vi "Test Serial.vi"() -> ()   [LabVIEW 2015]
uses:
  <vilib>/eio/EIOMethodNode/EIOMethodNode.xnode
  <vilib>/rvi/eio/common/nirviEmuTemplateMethod_errors.vi
  RS485 In.ctl
  Port.ctl
panel:
  out "Output":T1={"Data"=[0, 0, 0, 0, 0, 0, 0, 0, 0, 0, 0, 0, 0, 0, 0, 0, 0, 0, 0, 0, 0, 0, 0, 0, 0, 0, 0, 0, 0, 0, 0, 0, 0, 0, 0, 0, 0, 0, 0, 0, 0, 0, 0, 0, 0, 0, 0, 0, 0, 0, 0, 0, 0, 0, 0, 0, 0, 0, 0, 0, 0, 0, 0, 0, 0, 0, 0, 0, 0, 0, 0, 0, 0, 0, 0, 0, 0, 0, 0, 0, 0, 0, 0, 0, 0, 0, 0, 0, 0, 0, 0, 0, 0, 0, 0, 0, 0, 0, 0, 0, 0, 0, 0, 0, 0, 0, 0, 0, 0, 0, 0, 0, 0, 0, 0, 0, 0, 0, 0, 0, 0, 0, 0, 0, 0, 0, 0, 0, 0, 0, 0, 0, 0, 0, 0, 0, 0, 0, 0, 0, 0, 0, 0, 0, 0, 0, 0, 0, 0, 0, 0, 0, 0, 0, 0, 0, 0, 0, 0, 0, 0, 0, 0, 0, 0, 0, 0, 0, 0, 0, 0, 0, 0, 0, 0, 0, 0, 0, 0, 0, 0, 0, 0, 0, 0, 0, 0, 0, 0, 0, 0, 0, 0, 0, 0, 0, 0, 0, 0, 0], "NumBytes"=0, "RS485_Cmd"=enum."Read", "Port"=enum."Port 1", "Timeout (ms)"=0, "New"=FALSE}
  in  "Input":T1={"Data"=[0, 0, 0, 0, 0, 0, 0, 0, 0, 0, 0, 0, 0, 0, 0, 0, 0, 0, 0, 0, 0, 0, 0, 0, 0, 0, 0, 0, 0, 0, 0, 0, 0, 0, 0, 0, 0, 0, 0, 0, 0, 0, 0, 0, 0, 0, 0, 0, 0, 0, 0, 0, 0, 0, 0, 0, 0, 0, 0, 0, 0, 0, 0, 0, 0, 0, 0, 0, 0, 0, 0, 0, 0, 0, 0, 0, 0, 0, 0, 0, 0, 0, 0, 0, 0, 0, 0, 0, 0, 0, 0, 0, 0, 0, 0, 0, 0, 0, 0, 0, 0, 0, 0, 0, 0, 0, 0, 0, 0, 0, 0, 0, 0, 0, 0, 0, 0, 0, 0, 0, 0, 0, 0, 0, 0, 0, 0, 0, 0, 0, 0, 0, 0, 0, 0, 0, 0, 0, 0, 0, 0, 0, 0, 0, 0, 0, 0, 0, 0, 0, 0, 0, 0, 0, 0, 0, 0, 0, 0, 0, 0, 0, 0, 0, 0, 0, 0, 0, 0, 0, 0, 0, 0, 0, 0, 0, 0, 0, 0, 0, 0, 0, 0, 0, 0, 0, 0, 0, 0, 0, 0, 0, 0, 0, 0, 0, 0, 0, 0, 0], "NumBytes"=0, "RS485_Cmd"=enum."Idle", "Port"=enum."Port 1", "Timeout (ms)"=0, "New"=FALSE}
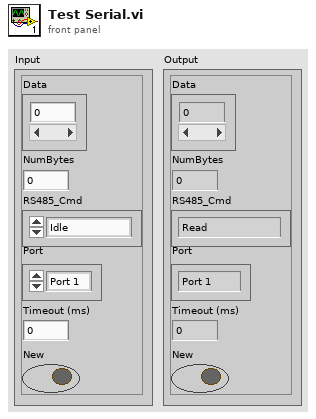
[diagram p1: front panel]
types:
  T1 = typedef "RS485 In.ctl" = cluster{"Data":u8[], "NumBytes":i32, "RS485_Cmd":enum8{"Read", "Write", "Idle"}, "Port":T2, "Timeout (ms)":i32, "New":bool}
  T2 = typedef "Port.ctl" = enum8{"Port 1", "Port 2", "Port 3", "Port 4", "None"}
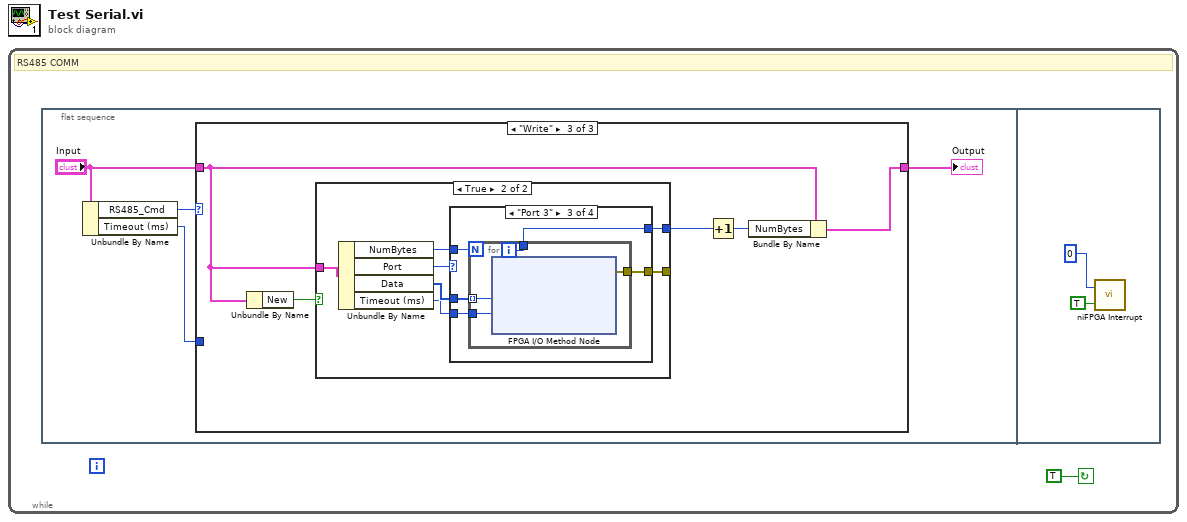
[diagram p0: block diagram]
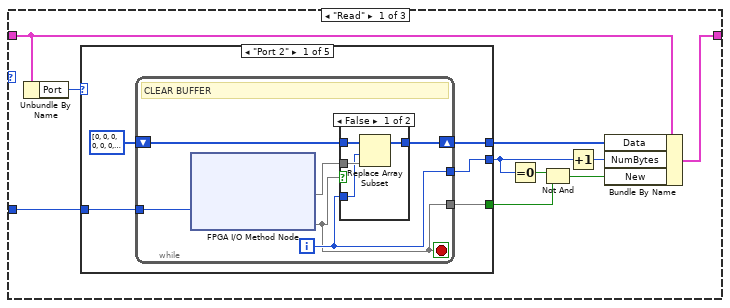
[diagram p2: hidden frame]
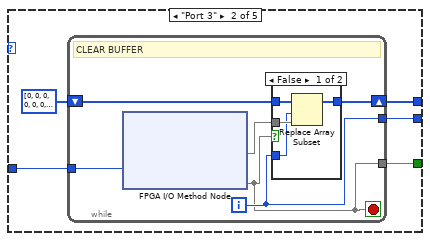
[diagram p4: hidden frame]
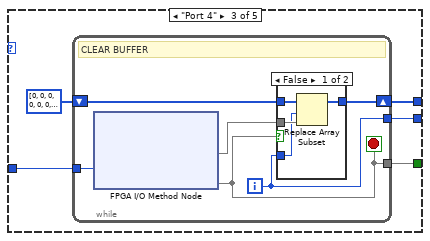
[diagram p6: hidden frame]
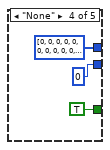
[diagram p8: hidden frame]
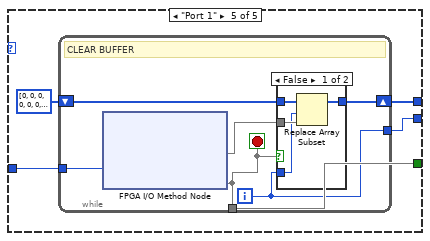
[diagram p9: hidden frame]
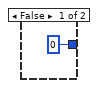
[diagram p12: hidden frame]
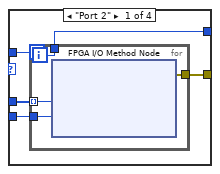
[diagram p13: hidden frame]
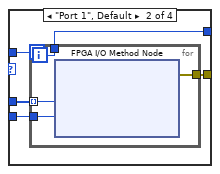
[diagram p14: hidden frame]
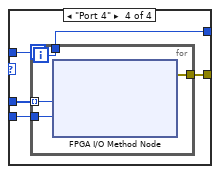
[diagram p15: hidden frame]
diagram:
  n1 = while {
    stop <- TRUE continue-if-true
    # "RS485 COMM"
    n2 = flat-sequence {
      frame #0 {
        n3 = Unbundle By Name("Input") -> ("RS485_Cmd"=w4:enum8{"Read", "Write", "Idle"}, "Timeout (ms)"=w3:i32)
        n4 = case shown="\"Write\"" w4 {
          tunnel: "Input" -> [w7 w83 w87]
          tunnel: [w6 w83 w86] -> w2
          tunnel: w3 -> [w8 _ _]
          frame "Read" {
            n5 = Unbundle By Name(w7) -> ("Port"=w15:T2)
            n6 = case shown="\"Port 2\"" w15 {
              tunnel: [w19 w35 w51 u8[] [0, 0, 0, 0, 0, 0, 0, 0, 0, 0, 0, 0, 0, 0, 0, 0, 0, 0, 0, 0, 0, 0, 0, 0, 0, 0, 0, 0, 0, 0, 0, 0, 0, 0, 0, 0, 0, 0, 0, 0, 0, 0, 0, 0, 0, 0, 0, 0, 0, 0, 0, 0, 0, 0, 0, 0, 0, 0, 0, 0, 0, 0, 0, 0, 0, 0, 0, 0, 0, 0, 0, 0, 0, 0, 0, 0, 0, 0, 0, 0, 0, 0, 0, 0, 0, 0, 0, 0, 0, 0, 0, 0, 0, 0, 0, 0, 0, 0, 0, 0, 0, 0, 0, 0, 0, 0, 0, 0, 0, 0, 0, 0, 0, 0, 0, 0, 0, 0, 0, 0, 0, 0, 0, 0, 0, 0, 0, 0, 0, 0, 0, 0, 0, 0, 0, 0, 0, 0, 0, 0, 0, 0, 0, 0, 0, 0, 0, 0, 0, 0, 0, 0, 0, 0, 0, 0, 0, 0, 0, 0, 0, 0, 0, 0, 0, 0, 0, 0, 0, 0, 0, 0, 0, 0, 0, 0, 0, 0, 0, 0, 0, 0, 0, 0, 0, 0, 0, 0, 0, 0, 0, 0, 0, 0, 0, 0, 0, 0, 0, 0] w70] -> w14
              tunnel: [w18 w34 w50 0 w69] -> w11
              tunnel: w8 -> [w17 w33 w49 _ w68]
              tunnel: [w16 w32 w48 TRUE ("Timed Out") w67] -> w10
              frame "Port 2" {
                n7 = while {
                  shift-right: [w25] -> w19
                  shift-left: u8[] [0, 0, 0, 0, 0, 0, 0, 0, 0, 0, 0, 0, 0, 0, 0, 0, 0, 0, 0, 0, 0, 0, 0, 0, 0, 0, 0, 0, 0, 0, 0, 0, 0, 0, 0, 0, 0, 0, 0, 0, 0, 0, 0, 0, 0, 0, 0, 0, 0, 0, 0, 0, 0, 0, 0, 0, 0, 0, 0, 0, 0, 0, 0, 0, 0, 0, 0, 0, 0, 0, 0, 0, 0, 0, 0, 0, 0, 0, 0, 0, 0, 0, 0, 0, 0, 0, 0, 0, 0, 0, 0, 0, 0, 0, 0, 0, 0, 0, 0, 0, 0, 0, 0, 0, 0, 0, 0, 0, 0, 0, 0, 0, 0, 0, 0, 0, 0, 0, 0, 0, 0, 0, 0, 0, 0, 0, 0, 0, 0, 0, 0, 0, 0, 0, 0, 0, 0, 0, 0, 0, 0, 0, 0, 0, 0, 0, 0, 0, 0, 0, 0, 0, 0, 0, 0, 0, 0, 0, 0, 0, 0, 0, 0, 0, 0, 0, 0, 0, 0, 0, 0, 0, 0, 0, 0, 0, 0, 0, 0, 0, 0, 0, 0, 0, 0, 0, 0, 0, 0, 0, 0, 0, 0, 0, 0, 0, 0, 0, 0, 0] -> [w26]
                  tunnel: [w24] -> w18
                  tunnel: w17 -> [w22]
                  tunnel: [w21] -> w16
                  i -> [w24]
                  stop <- w21 stop-if-true
                  # "CLEAR BUFFER"
                  n8 = xnode "FPGA I/O Method Node"("Timeout (ms)"=w22) -> ("Data"=w23, "Timed Out"=w21)  [unwired: 1 in, 1 out]
                  n9 = case shown="False" w21 {
                    tunnel: w26 -> [w30 w31]
                    tunnel: [w27 w31] -> w25
                    tunnel: w23 -> [w29 _]
                    tunnel: w24 -> [w28 _]
                    frame False {
                      n10 = Replace Array Subset(array=w30, new element=w29, index=w28) -> (w27:u8[])
                    }
                    frame True {
                    }
                  }
                }
              }
              frame "Port 3" {
                n11 = while {
                  shift-right: [w41] -> w35
                  shift-left: u8[] [0, 0, 0, 0, 0, 0, 0, 0, 0, 0, 0, 0, 0, 0, 0, 0, 0, 0, 0, 0, 0, 0, 0, 0, 0, 0, 0, 0, 0, 0, 0, 0, 0, 0, 0, 0, 0, 0, 0, 0, 0, 0, 0, 0, 0, 0, 0, 0, 0, 0, 0, 0, 0, 0, 0, 0, 0, 0, 0, 0, 0, 0, 0, 0, 0, 0, 0, 0, 0, 0, 0, 0, 0, 0, 0, 0, 0, 0, 0, 0, 0, 0, 0, 0, 0, 0, 0, 0, 0, 0, 0, 0, 0, 0, 0, 0, 0, 0, 0, 0, 0, 0, 0, 0, 0, 0, 0, 0, 0, 0, 0, 0, 0, 0, 0, 0, 0, 0, 0, 0, 0, 0, 0, 0, 0, 0, 0, 0, 0, 0, 0, 0, 0, 0, 0, 0, 0, 0, 0, 0, 0, 0, 0, 0, 0, 0, 0, 0, 0, 0, 0, 0, 0, 0, 0, 0, 0, 0, 0, 0, 0, 0, 0, 0, 0, 0, 0, 0, 0, 0, 0, 0, 0, 0, 0, 0, 0, 0, 0, 0, 0, 0, 0, 0, 0, 0, 0, 0, 0, 0, 0, 0, 0, 0, 0, 0, 0, 0, 0, 0] -> [w42]
                  tunnel: [w40] -> w34
                  tunnel: w33 -> [w38]
                  tunnel: [w37] -> w32
                  i -> [w40]
                  stop <- w37 stop-if-true
                  # "CLEAR BUFFER"
                  n12 = xnode "FPGA I/O Method Node"("Timeout (ms)"=w38) -> ("Data"=w39, "Timed Out"=w37)  [unwired: 1 in, 1 out]
                  n13 = case shown="False" w37 {
                    tunnel: w42 -> [w46 w47]
                    tunnel: [w43 w47] -> w41
                    tunnel: w39 -> [w45 _]
                    tunnel: w40 -> [w44 _]
                    frame False {
                      n14 = Replace Array Subset(array=w46, new element=w45, index=w44) -> (w43:u8[])
                    }
                    frame True {
                    }
                  }
                }
              }
              frame "Port 4" {
                n15 = while {
                  shift-right: [w57] -> w51
                  shift-left: u8[] [0, 0, 0, 0, 0, 0, 0, 0, 0, 0, 0, 0, 0, 0, 0, 0, 0, 0, 0, 0, 0, 0, 0, 0, 0, 0, 0, 0, 0, 0, 0, 0, 0, 0, 0, 0, 0, 0, 0, 0, 0, 0, 0, 0, 0, 0, 0, 0, 0, 0, 0, 0, 0, 0, 0, 0, 0, 0, 0, 0, 0, 0, 0, 0, 0, 0, 0, 0, 0, 0, 0, 0, 0, 0, 0, 0, 0, 0, 0, 0, 0, 0, 0, 0, 0, 0, 0, 0, 0, 0, 0, 0, 0, 0, 0, 0, 0, 0, 0, 0, 0, 0, 0, 0, 0, 0, 0, 0, 0, 0, 0, 0, 0, 0, 0, 0, 0, 0, 0, 0, 0, 0, 0, 0, 0, 0, 0, 0, 0, 0, 0, 0, 0, 0, 0, 0, 0, 0, 0, 0, 0, 0, 0, 0, 0, 0, 0, 0, 0, 0, 0, 0, 0, 0, 0, 0, 0, 0, 0, 0, 0, 0, 0, 0, 0, 0, 0, 0, 0, 0, 0, 0, 0, 0, 0, 0, 0, 0, 0, 0, 0, 0, 0, 0, 0, 0, 0, 0, 0, 0, 0, 0, 0, 0, 0, 0, 0, 0, 0, 0] -> [w58]
                  tunnel: [w56] -> w50
                  tunnel: w49 -> [w54]
                  tunnel: [w53] -> w48
                  i -> [w56]
                  stop <- w53 stop-if-true
                  # "CLEAR BUFFER"
                  n16 = xnode "FPGA I/O Method Node"("Timeout (ms)"=w54) -> ("Data"=w55, "Timed Out"=w53)  [unwired: 1 in, 1 out]
                  n17 = case shown="False" w53 {
                    tunnel: w58 -> [w62 w63]
                    tunnel: [w59 w63] -> w57
                    tunnel: w55 -> [w61 _]
                    tunnel: w56 -> [w60 _]
                    frame False {
                      n18 = Replace Array Subset(array=w62, new element=w61, index=w60) -> (w59:u8[])
                    }
                    frame True {
                    }
                  }
                }
              }
              frame "None" {
              }
              frame "Port 1" {
                n19 = while {
                  shift-right: [w76] -> w70
                  shift-left: u8[] [0, 0, 0, 0, 0, 0, 0, 0, 0, 0, 0, 0, 0, 0, 0, 0, 0, 0, 0, 0, 0, 0, 0, 0, 0, 0, 0, 0, 0, 0, 0, 0, 0, 0, 0, 0, 0, 0, 0, 0, 0, 0, 0, 0, 0, 0, 0, 0, 0, 0, 0, 0, 0, 0, 0, 0, 0, 0, 0, 0, 0, 0, 0, 0, 0, 0, 0, 0, 0, 0, 0, 0, 0, 0, 0, 0, 0, 0, 0, 0, 0, 0, 0, 0, 0, 0, 0, 0, 0, 0, 0, 0, 0, 0, 0, 0, 0, 0, 0, 0, 0, 0, 0, 0, 0, 0, 0, 0, 0, 0, 0, 0, 0, 0, 0, 0, 0, 0, 0, 0, 0, 0, 0, 0, 0, 0, 0, 0, 0, 0, 0, 0, 0, 0, 0, 0, 0, 0, 0, 0, 0, 0, 0, 0, 0, 0, 0, 0, 0, 0, 0, 0, 0, 0, 0, 0, 0, 0, 0, 0, 0, 0, 0, 0, 0, 0, 0, 0, 0, 0, 0, 0, 0, 0, 0, 0, 0, 0, 0, 0, 0, 0, 0, 0, 0, 0, 0, 0, 0, 0, 0, 0, 0, 0, 0, 0, 0, 0, 0, 0] -> [w77]
                  tunnel: [w75] -> w69
                  tunnel: w68 -> [w73]
                  tunnel: [w72] -> w67
                  i -> [w75]
                  stop <- w72 stop-if-true
                  # "CLEAR BUFFER"
                  n20 = xnode "FPGA I/O Method Node"("Timeout (ms)"=w73) -> ("Data"=w74, "Timed Out"=w72)  [unwired: 1 in, 1 out]
                  n21 = case shown="False" w72 {
                    tunnel: w77 -> [w81 w82]
                    tunnel: [w78 w82] -> w76
                    tunnel: w74 -> [w80 _]
                    tunnel: w75 -> [w79 _]
                    frame False {
                      n22 = Replace Array Subset(array=w81, new element=w80, index=w79) -> (w78:u8[])
                    }
                    frame True {
                    }
                  }
                }
              }
            }
            n23 = Equal To 0?(x=w11) -> (x = 0?=w12:bool)
            n24 = Not And(1:w10, 2:w12) -> (0:w9:bool)
            n25 = Increment(x=w11) -> (x+1=w13:i32)
            n26 = Bundle By Name(cluster=w7, "Data"=w14, "NumBytes"=w13, "New"=w9) -> (w6:T1)
          }
          frame "Idle", Default {
          }
          frame "Write" {
            n27 = Unbundle By Name(w87) -> ("New"=w88:bool)
            n28 = case shown="True" w88 {
              tunnel: w87 -> [_ w96]
              tunnel: [_ w92] -> _
              tunnel: [0 w90] -> w85
              frame False {
              }
              frame True {
                n29 = Unbundle By Name(w96) -> ("NumBytes"=w95:i32, "Port"=w93:T2, "Data"=w94:u8[], "Timeout (ms)"=w91:i32)
                n30 = case shown="\"Port 3\"" w93 {
                  tunnel: w95 -> [w101 w110 w119 w128]
                  tunnel: w94 -> [w100 w109 w118 w127]
                  tunnel: [w99 w108 w117 w126] -> w92
                  tunnel: w91 -> [w98 w107 w116 w125]
                  tunnel: [w97 w106 w115 w124] -> w90
                  frame "Port 2" {
                    n31 = for {
                      N: w101 -> [_]
                      tunnel: w100 -> [w103] mode=indexing
                      tunnel: w98 -> [w105]
                      tunnel: [w104] -> w99
                      tunnel: [w102] -> w97
                      i -> [w102]
                      n32 = xnode "FPGA I/O Method Node"("Data"=w103, "Timeout (ms)"=w105) -> ("error out"=w104:errorcluster)  [unwired: 2 in, 2 out]
                    }
                  }
                  frame "Port 1", Default {
                    n33 = for {
                      N: w110 -> [_]
                      tunnel: w109 -> [w114] mode=indexing
                      tunnel: w107 -> [w113]
                      tunnel: [w112] -> w108
                      tunnel: [w111] -> w106
                      i -> [w111]
                      n34 = xnode "FPGA I/O Method Node"("Data"=w114, "Timeout (ms)"=w113) -> ("error out"=w112:errorcluster)  [unwired: 2 in, 2 out]
                    }
                  }
                  frame "Port 3" {
                    n35 = for {
                      N: w119 -> [_]
                      tunnel: w118 -> [w123] mode=indexing
                      tunnel: w116 -> [w122]
                      tunnel: [w121] -> w117
                      tunnel: [w120] -> w115
                      i -> [w120]
                      n36 = xnode "FPGA I/O Method Node"("Data"=w123, "Timeout (ms)"=w122) -> ("error out"=w121:errorcluster)  [unwired: 2 in, 2 out]
                    }
                  }
                  frame "Port 4" {
                    n37 = for {
                      N: w128 -> [_]
                      tunnel: w127 -> [w132] mode=indexing
                      tunnel: w125 -> [w131]
                      tunnel: [w130] -> w126
                      tunnel: [w129] -> w124
                      i -> [w129]
                      n38 = xnode "FPGA I/O Method Node"("Data"=w132, "Timeout (ms)"=w131) -> ("error out"=w130:errorcluster)  [unwired: 2 in, 2 out]
                    }
                  }
                }
              }
            }
            n39 = Increment(x=w85) -> (x+1=w84:i32)
            n40 = Bundle By Name(cluster=w87, "NumBytes"=w84) -> (w86:T1)
          }
        }
        "Output" <- w2
      }
      frame #1 {
        n41 = call <vilib>:"niFPGA Interrupt.vi"("Wait Until Cleared (F)"=TRUE, "IRQ Number (0)"=u8 0) -> ()  [unwired: 1 in]
      }
    }
  }
